vi "rfmapper.vi"() -> ()   [LabVIEW 2011]
uses:
  <instrlib>/niHWS/nihws.llb/niHWS Open File Permissions ID.ctl
  <vilib>/vision/Image Controls.llb/IMAQ Rounding Mode.ctl
  <vilib>/DAQmx/write.llb/DAQmx Write (Analog Wfm 1Chan NSamp).vi
  <vilib>/DAQmx/read.llb/DAQmx Read (Analog 1D Wfm NChan NSamp).vi
  <vilib>/DAQmx/create/channels.llb/DAQmx Create Channel (AO-Voltage-Basic).vi
  <vilib>/DAQmx/configure/timing.llb/DAQmx Timing (Sample Clock).vi
  <vilib>/DAQmx/create/channels.llb/DAQmx Create Channel (AI-Voltage-Basic).vi
  <instrlib>/niHWS/nihws.llb/niHWS Write Analog DBL.vi
  <vilib>/DAQmx/miscellaneous.llb/DAQmx Fill In Error Info.vi
  <vilib>/Analysis/2dsp.llb/1D Cross Correlation (DBL).vi
  <vilib>/Analysis/baseanly.llb/Real Outer Product.vi
  <instrlib>/niHWS/nihws.llb/niHWS Write Analog WDT.vi
  <vilib>/Analysis/NI_AALBase.lvlib
  <vilib>/Analysis/NI_AALPro.lvlib
  <vilib>/ptbypt/NI_PtbyPt.lvlib
  <vilib>/vision/NI_Vision_Development_Module.lvlib
  C:/Program Files/National Instruments/LabVIEW 2011/resource/objmgr/IMAQImage.rc
  C:/Program Files/National Instruments/LabVIEW 2011/resource/objmgr/daqmx.rc
panel:
  in  "Audio Channel":dbl
  out "Waveform Chart 4":dynamicdata(graph)
  in  "audio gain":dbl(knob) scale=0.0..1000000000.0
  in  "Image Size\nX                  Y":dbl[][](array[numeric])=[[0.02, 0.0], [0.99, 0.55]]
  in  "Threshold":dbl=0.3
  in  "Auto\nThreshold":bool
  in  "Recording Path":path
  in  "Record":bool
  in  "Recording channels":tag
  in  "Auto \nDelay":bool
  in  "90-270 delay":dbl
  in  "0-180 delay":dbl
  in  "Ref. \nperiod":dbl=3.0 caption="Time Target (s)"
  out "Count":bool
  out "Wait":bool
  in  "Filter":bool=TRUE
  in  "Binarize Map":bool
  in  "Clear 270":bool
  in  "Clear 180":bool
  in  "Clear 90":bool
  in  "Clear 0":bool
  out "Screen":T1(plugin-control)
  out "Collected Signals 3":dbl[][](graph) caption="Collected Signals"
  out "Waveform Graph":dbl[][](graph)
  out "signal size":i32
  out "270":i32[](array[numeric])
  out "90":i32[](array[numeric])
  out "180":i32[](array[numeric])
  out "0":i32[](array[numeric])
  in  "Bar Direction":u16(ring)=4 items=["270"=3, "90"=2, "180"=1, "0"=0]
  out "Collected Signals 2":dbl[][](graph) caption="Collected Signals"
  out "Waveform Chart 3":dynamicdata(graph)
  out "Collected Signals":dbl[](graph)
  out "Trigger":bool
  out "Waveform Chart":waveform(dbl)(graph)
  in  "stop":bool
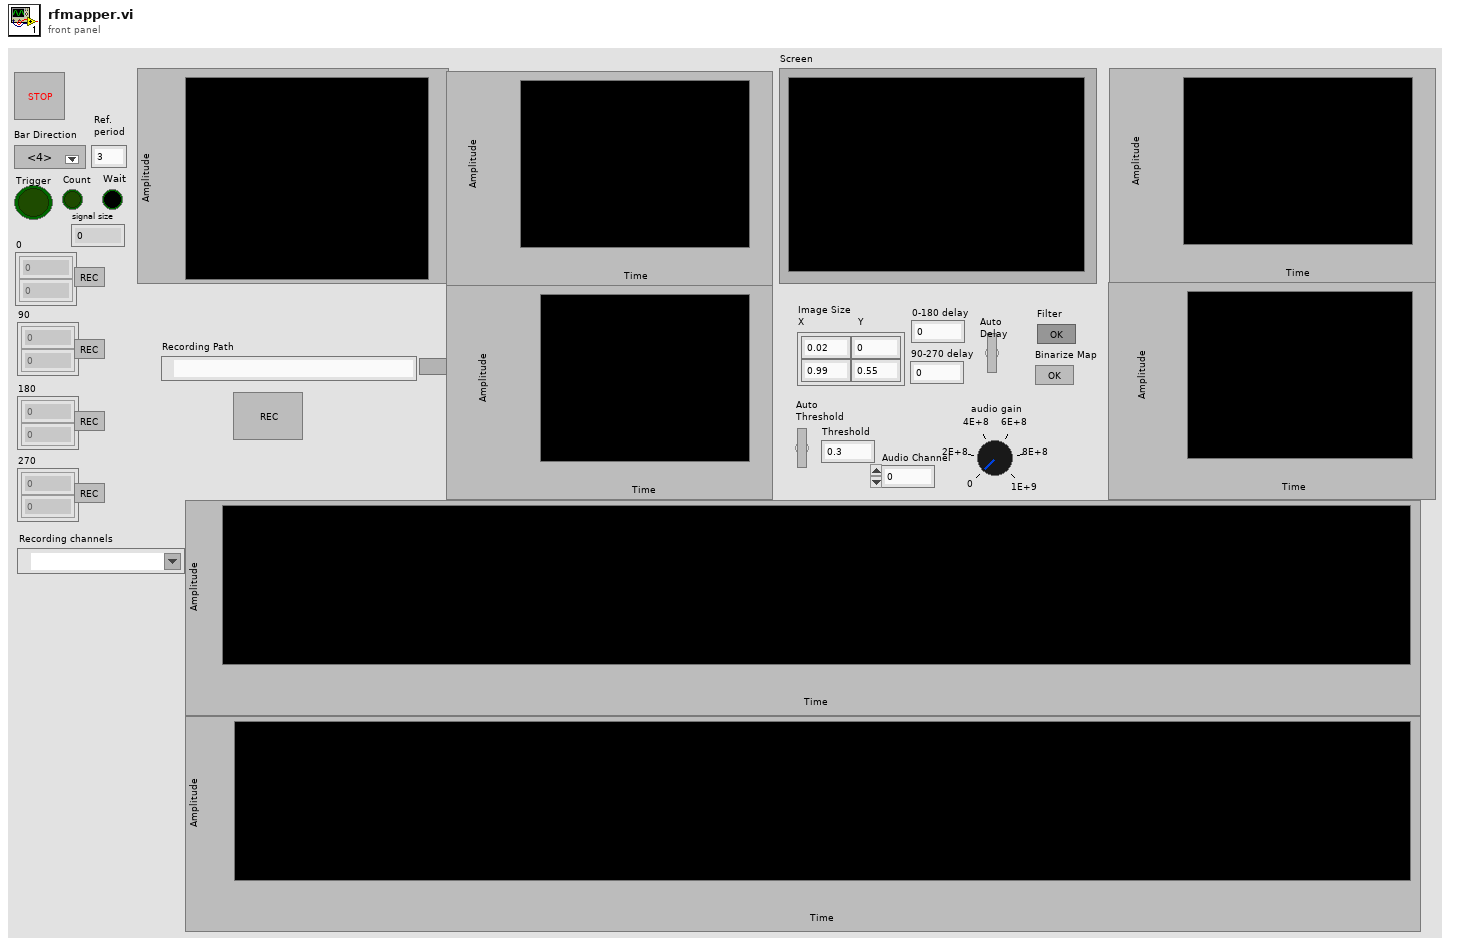
[diagram p1: front panel]
types:
  T1 = typedef "IMAQ Image.ctl" = refnum<image>
  T2 = typedef "niHWS Open File Permissions ID.ctl" = enum32{"Read Only", "Read/Write Existing", "Read/Write/Create New", "Read/Write/Create New Always"}
  T3 = typedef "Image Type" = u32
  T4 = typedef "IMAQ Rounding Mode.ctl" = enum16{"Optimize", "Truncate"}
  T5 = typedef "NI_Matrix.lvlib/RealMatrix.ctl" = dbl[][]
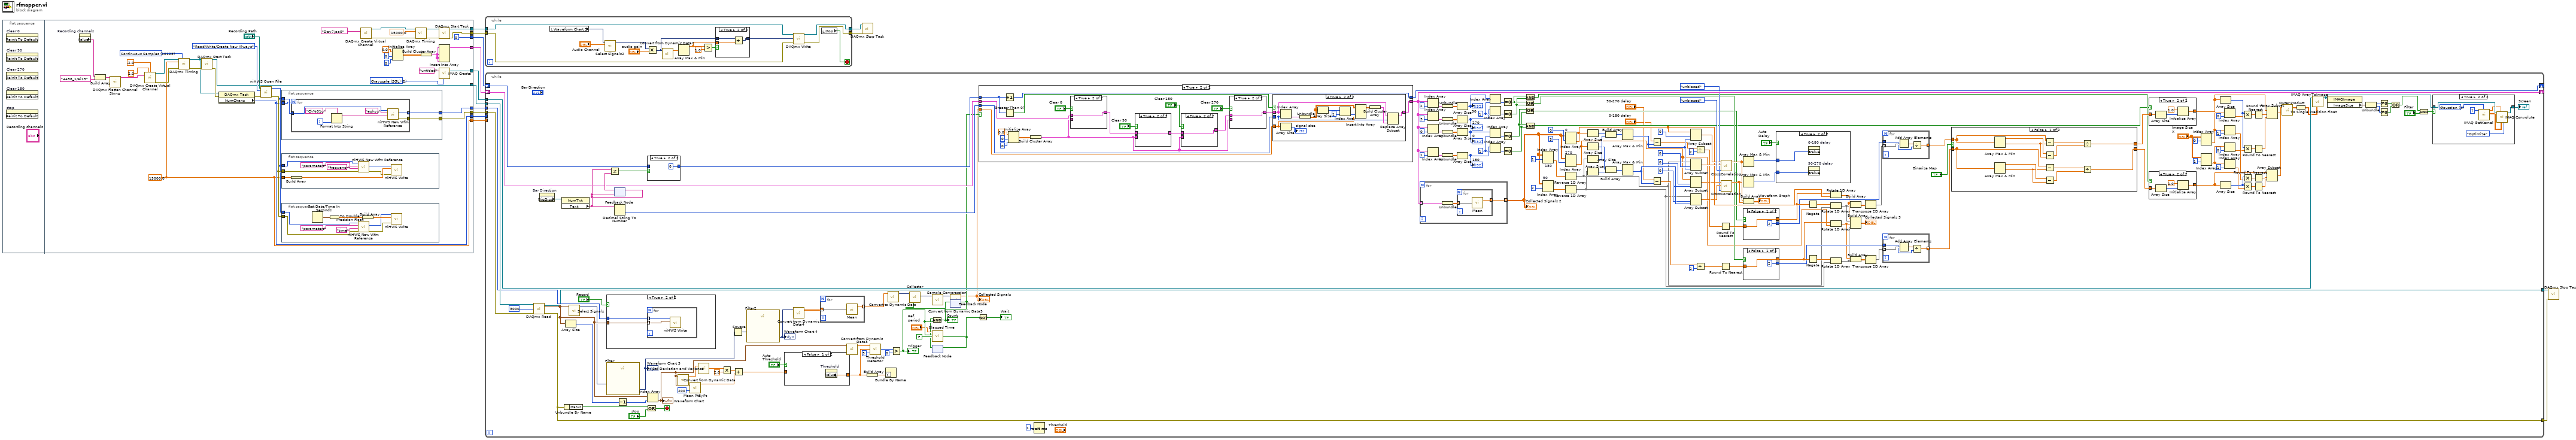
[diagram p0: block diagram]
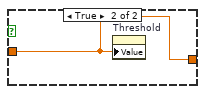
[diagram p3: hidden frame]
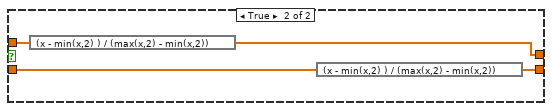
[diagram p7: hidden frame]
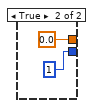
[diagram p10: hidden frame]
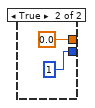
[diagram p11: hidden frame]
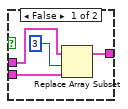
[diagram p14: hidden frame]
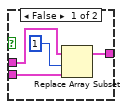
[diagram p15: hidden frame]
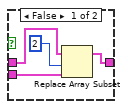
[diagram p16: hidden frame]
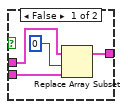
[diagram p17: hidden frame]
diagram:
  n1 = flat-sequence {
    tunnel: [0] -> w14
    tunnel: [w49] -> w13
    tunnel: [w47] -> w12
    tunnel: [w31] -> w11
    tunnel: [w30] -> w10
    tunnel: [w29] -> w9
    tunnel: [w28] -> w8
    tunnel: [w27] -> w5
    tunnel: [w16] -> w2
    tunnel: [w15] -> w1
    frame #0 {
      n2 = invoke on="Clear 0" class="Bool (strict)" method="Reinit To Default"() -> ()  [unwired: 3 in, 3 out]
      n3 = invoke on="Clear 90" class="Bool (strict)" method="Reinit To Default"() -> ()  [unwired: 3 in, 3 out]
      n4 = invoke on="Clear 270" class="Bool (strict)" method="Reinit To Default"() -> ()  [unwired: 3 in, 3 out]
      n5 = invoke on="Clear 180" class="Bool (strict)" method="Reinit To Default"() -> ()  [unwired: 3 in, 3 out]
      n6 = invoke on="stop" class="Bool (strict)" method="Reinit To Default"() -> ()  [unwired: 3 in, 3 out]
    }
    frame #1 {
      w41 = 10123 items=["Finite Samples"=10178, "Continuous Samples"=10123, "Hardware Timed Single Point"=12522] ("sample mode")
      w27 = 15000.0 ("rate")
      w45 = T3 2 items=["Grayscale (U8)", "Grayscale (I16)", "Grayscale (SGL)", "Complex (CSG)", "RGB (U32)", "HSL (U32)", "RGB (U64)", "Grayscale (U16)"] ("Image Type")
      n7 = property on="Recording channels" class="DAQmxName"() -> ("Value"=w24:string)  [unwired: 2 in, 2 out]
      n8 = Build Array(w24, tag "4498_1/ai15" ("Recording channels 3")) -> (w26:string[])
      n9 = call <vilib>:"DAQmx Flatten Channel String.vi"("names in"=w26) -> ("names out"=w23:string)  [unwired: 13 in, 1 out]
      n10 = call-poly <vilib>:"DAQmx Create Virtual Channel.vi"("maximum value"=2.0, "minimum value"=-2.0, "physical channels"=w23) -> ("task out"=w42:refnum<k21>, "error out"=w40:errorcluster)  [unwired: 11 in]
      n11 = call-poly <vilib>:"DAQmx Timing.vi"("task/channels in"=w42, "sample mode"=w41, "rate"=w27, "error in"=w40) -> ("task out"=w37:refnum<k21>, "error out"=w39:errorcluster)  [unwired: 10 in]
      n12 = call <vilib>:"DAQmx Start Task.vi"("task/channels in"=w37, "error in"=w39) -> ("task out"=w31:refnum<k21>, "error out"=w38:errorcluster)  [unwired: 12 in]
      n13 = property class="DAQmx Task"(reference=w37, error in=w38) -> (error out=w34:errorcluster, "NumChans"=w30:u32)  [unwired: 1 out]
      n14 = call <instrlib>:"niHWS Open File.vi"("error in (no error)"=w34, "permissions (0:read only)"=niHWS_Open_File_Permissions_ID."Read/Write/Create New Always", "file path"="Recording Path") -> ("error out"=w33:errorcluster, "file handle"=w32:u32)  [unwired: 7 in]
      n15 = flat-sequence {
        tunnel: w30 -> [w74]
        tunnel: w32 -> [w75]
        tunnel: [w73] -> w28
        tunnel: [w72] -> w29
        frame #0 {
          n16 = for {
            N: w74 -> [_]
            tunnel: [w77] -> w73 mode=indexing
            tunnel: [w76] -> w72
            tunnel: w75 -> [w82]
            i -> [w80]
            n17 = Format Into String(format string="Ch%01u", w80) -> (resulting string=w78:string)  [unwired: 2 in, 1 out]
            n18 = call <instrlib>:"niHWS New Wfm Reference.vi"("waveform name (empty)"=w78, "group name (empty)"="ephys", "file handle in"=w82) -> ("error out"=w76:errorcluster, "waveform reference"=w77:u32)  [unwired: 6 in, 1 out]
          }
        }
      }
      n19 = flat-sequence {
        tunnel: w27 -> [w67]
        tunnel: w33 -> [w66]
        tunnel: w32 -> [w65]
        frame #0 {
          n20 = Build Array(w67) -> (w68:dbl[])
          n21 = call <instrlib>:"niHWS New Wfm Reference.vi"("error in (no error)"=w66, "waveform name (empty)"="frequency" ("group name (empty)"), "group name (empty)"="parameters", "file handle in"=w65) -> ("error out"=w64:errorcluster, "waveform reference"=w71:u32)  [unwired: 5 in, 1 out]
          n22 = call-poly <instrlib>:"niHWS Write.vi"("error in (no error)"=w64, "data"=w68, "waveform reference in"=w71) -> ()  [unwired: 7 in, 2 out]
        }
      }
      n23 = flat-sequence {
        tunnel: w33 -> [w63]
        tunnel: w32 -> [w62]
        frame #0 {
          n24 = Get Date/Time In Seconds() -> (seconds since 1Jan1904=w61:timestamp)
          n25 = To Double Precision Float(number=w61) -> (double precision float=w60:dbl)
          n26 = call <instrlib>:"niHWS New Wfm Reference.vi"("error in (no error)"=w63, "waveform name (empty)"="time" ("group name (empty)"), "group name (empty)"="parameters", "file handle in"=w62) -> ("error out"=w55:errorcluster, "waveform reference"=w56:u32)  [unwired: 5 in, 1 out]
          n27 = Build Array(w60) -> (w59:dbl[])
          n28 = call-poly <instrlib>:"niHWS Write.vi"("error in (no error)"=w55, "data"=w59, "waveform reference in"=w56) -> ()  [unwired: 7 in, 2 out]
        }
      }
      n29 = call-poly <vilib>:"DAQmx Create Virtual Channel.vi"("physical channels"=tag "Dev7/ao0") -> ("task out"=w21:refnum<k21>, "error out"=w18:errorcluster)  [unwired: 13 in]
      n30 = Initialize Array(0.0, 0, 0) -> (w53:dbl[][])
      n31 = call-poly <vilib>:"DAQmx Timing.vi"("task/channels in"=w21, "rate"=15000.0, "error in"=w18) -> ("task out"=w19:refnum<k21>, "error out"=w17:errorcluster)  [unwired: 11 in]
      n32 = Build Cluster Array(w53) -> (w48:cluster{dbl[][]}[])
      n33 = call <vilib>:"DAQmx Start Task.vi"("task/channels in"=w19, "error in"=w17) -> ("task out"=w16:refnum<k21>, "error out"=w15:errorcluster)  [unwired: 12 in]
      n34 = Insert Into Array(array=w48, new element #1=w48, new element #2=w48, new element #3=w48) -> (w49:cluster{dbl[][]}[])  [unwired: 1 in]
      n35 = call "IMAQ Create"("Image Name"="untitled", "Image Type"=w45) -> ("New Image"=w47:T1)  [unwired: 3 in, 1 out]
    }
  }
  n36 = while {
    tunnel: [w96] -> w4
    tunnel: [w95] -> w3
    tunnel: w2 -> [w94]
    tunnel: w1 -> [w93]
    stop <- w97 stop-if-true
    n37 = local read "Waveform Chart 3"() -> (w85:dynamicdata)
    n38 = call "Select Signals2"("Selector Input"="Audio Channel", "Signals"=w85) -> ("Signal Out"=w83:dynamicdata)  [unwired: 8 in, 1 out]
    n39 = Multiply(x=w83, y="audio gain") -> (x*y=w88:dynamicdata)
    n40 = call "Convert from Dynamic Data2"("Dynamic Data Type"=w88) -> ("Array"=w91:dbl[])  [unwired: 3 in]
    n41 = Array Max & Min(array=w91) -> (max value=w86:dbl)  [unwired: 3 out]
    n42 = Greater?(x=w86, y=1.0) -> (0:w89:bool)
    n43 = case shown="True" w89 {
      tunnel: w88 -> [w98 w101]
      tunnel: [w98 w99] -> w87
      tunnel: w86 -> [_ w100]
      frame False {
      }
      frame True {
        n44 = Divide(x=w101, y=w100) -> (x/y=w99:dynamicdata)
      }
    }
    n45 = call-poly <vilib>:"DAQmx Write.vi"("task/channels in"=w94, "data"=w87, "error in"=w93) -> ("task out"=w96:refnum<k21>, "error out"=w95:errorcluster)  [unwired: 10 in, 1 out]
    n46 = local read "stop"() -> (w97:bool)
  }
  n47 = while {
    shift-right: [w285] -> _
    shift-left: w14 -> [w264]
    shift-right: [w271] -> _
    shift-left: w13 -> [w201]
    tunnel: w12 -> [w209]
    tunnel: w11 -> [w164]
    tunnel: w10 -> [_]
    tunnel: w9 -> [w165]
    tunnel: w8 -> [w163]
    tunnel: [w158] -> w7
    tunnel: [w157] -> w6
    tunnel: w5 -> [_]
    stop <- w159 stop-if-true
    w220 = 1 ("index")
    w227 = 1 ("index")
    n48 = call-poly <vilib>:"DAQmx Read.vi"("task/channels in"=w164, "number of samples per channel"=3000, "error in"=w165) -> ("task out"=w158:refnum<k21>, "data"=w129:waveform(dbl)[], "error out"=w157:errorcluster)  [unwired: 10 in]
    n49 = property on="Bar Direction" class="Ring (strict)"() -> ("DigDisp"=w284:refnum<vi>)  [unwired: 2 in, 2 out]
    n50 = property class="NumTxt"(reference=w284) -> ("Text"=w266:string)  [unwired: 1 in, 2 out]
    n51 = Unbundle By Name(w157) -> ("status"=w161:bool)
    n52 = Array Size(array=w129) -> (size(s)=w131:i32)
    n53 = call "Select Signals"("Signals"=w129) -> ("Signal Out"=w124:dynamicdata)  [unwired: 9 in, 1 out]
    n54 = case shown="True" "Record" {
      tunnel: w129 -> [_ w299]
      tunnel: w163 -> [_ w298]
      frame False {
      }
      frame True {
        n55 = for {
          tunnel: w299 -> [w301] mode=indexing
          tunnel: w298 -> [w300] mode=indexing
          n56 = call-poly <instrlib>:"niHWS Write.vi"("analog waveform"=w301, "waveform reference in"=w300) -> ()  [unwired: 8 in, 2 out]
        }
      }
    }
    n57 = call "Filter"("Signal"=w124) -> ("Filtered Signal"=w102:dynamicdata)  [unwired: 9 in, 1 out]
    "Waveform Chart 3" <- w102
    n58 = feedback-in #1(w266) -> ()
    n59 = feedback #1(w266) -> (w265:string)
    n60 = Not Equal?(x=w266, y=w265) -> (x != y?=w262:bool)
    n61 = Decimal String To Number(string=w266) -> (number=w270:i32)  [unwired: 2 in, 1 out]
    n62 = Decrement(x=w131) -> (x-1=w130:i32)
    n63 = Or(x=w161, y="stop") -> (x .or. y?=w159:bool)
    n64 = case shown="True" w262 {
      tunnel: w264 -> [w354 _]
      tunnel: [w354 0] -> w263
      frame False {
      }
      frame True {
      }
    }
    n65 = Index Array(array=w129, index=w130) -> (element=w123:waveform(dbl))
    "Waveform Chart" <- w123
    n66 = call "Convert from Dynamic Data"("Dynamic Data Type"=w123) -> ("Array"=w292:dbl[])  [unwired: 3 in]
    n67 = call <vilib>:"Mean PtByPt.vi"("x"=w123, "sample length"=200) -> ("mean"=w287:dbl)  [unwired: 2 in, 1 out]
    n68 = call <vilib>:"Std Deviation and Variance.vi"("X"=w292) -> ("standard deviation"=w291:dbl)  [unwired: 1 in, 2 out]
    n69 = Multiply(x=w291, y=2.0) -> (x*y=w288:dbl)
    n70 = Square(x=w102) -> (x^2=w104:dynamicdata)
    n71 = Add(x=w288, y=w287) -> (x+y=w152:dbl)
    n72 = call "Filter2"("Signal"=w104) -> ("Filtered Signal"=w103:dynamicdata)  [unwired: 9 in, 1 out]
    "Waveform Chart 4" <- w103
    n73 = case shown="False" "Auto\nThreshold" {
      tunnel: w152 -> [_ w297]
      tunnel: [w296 w297] -> w151
      frame False {
        n74 = property on="Threshold" class="DigNum (strict)"() -> ("Value"=w296:dbl)  [unwired: 2 in, 2 out]
      }
      frame True {
        n75 = property on="Threshold" class="DigNum (strict)"("Value"=w297) -> ()  [unwired: 2 in, 2 out]
      }
    }
    n76 = call "Convert from Dynamic Data4"("Dynamic Data Type"=w103) -> ("Array"=w128:dbl[][])  [unwired: 3 in]
    n77 = for {
      tunnel: w128 -> [w295] mode=indexing
      tunnel: [w294] -> w127 mode=indexing
      n78 = call <vilib>:"Mean.vi"("X"=w295) -> ("mean"=w294:dbl)  [unwired: 1 out]
    }
    n79 = call "Convert from Dynamic Data3"("Dynamic Data Type"=w123) -> ("Array"=w290:dbl[])  [unwired: 3 in]
    n80 = Build Array(w151) -> (w150:dbl[])
    n81 = call <vilib>:"Threshold Detector.vi"("width"=3, "threshold"=w151, "X"=w290) -> ("count"=w286:i32)  [unwired: 2 out]
    n82 = Bundle By Name("Y"=w150) -> ()  [unwired: 1 in, 1 out]
    n83 = call "Convert to Dynamic Data"("Array"=w127) -> ("Dynamic Data Type"=w126:dynamicdata)  [unwired: 3 in]
    n84 = Greater?(x=w286, y=0) -> (0:w177:bool)
    "Trigger" <- w177
    n85 = call "Elapsed Time"("Time Target (s)"="Ref. \nperiod", "Reset"=w177, "Auto Reset"=FALSE) -> ("Time has Elapsed"=w173:bool)  [unwired: 9 in, 7 out]
    n86 = feedback-in #2(w173) -> ()
    n87 = feedback #2() -> (w174:bool)  [unwired: 1 in]
    n88 = And(x=w174, y=w177) -> (x .and. y?=w133:bool)
    "Count" <- w133
    n89 = feedback-in #3(w133) -> ()
    n90 = feedback #3() -> (w132:bool)  [unwired: 1 in]
    n91 = call "Collector"("Reset"=w132, "Signals"=w126) -> ("Collected Signals"=w106:dynamicdata)  [unwired: 8 in, 1 out]
    n92 = call "Sample Compression"("Signals"=w106) -> ("Mean"=w105:dynamicdata)  [unwired: 8 in, 2 out]
    n93 = call "Convert from Dynamic Data5"("Dynamic Data Type"=w105) -> ("Array"=w125:dbl[])  [unwired: 3 in]
    "Collected Signals" <- w125
    n94 = Not(x=w173) -> (.not. x?=→"Wait":bool)
    n95 = case shown="True" w133 {
      tunnel: w263 -> [w362 w379]
      tunnel: [w362 w382] -> w285
      tunnel: w201 -> [w361 w373]
      tunnel: w125 -> [_ w363]
      tunnel: [w361 w381] -> w271
      tunnel: w270 -> [_ w380]
      frame False {
      }
      frame True {
        n96 = Increment(x=w379) -> (x+1=w382:i32)
        n97 = Greater Than 0?(x=w379) -> (x > 0?=w378:bool)
        n98 = Initialize Array(0.0, 0, 0) -> (w377:dbl[][])
        n99 = Build Cluster Array(w377) -> (w372:cluster{dbl[][]}[])
        n100 = case shown="True" "Clear 0" {
          tunnel: w373 -> [w400 w402]
          tunnel: [w398 w402] -> w364
          tunnel: w372 -> [w399 _]
          frame False {
            n101 = Replace Array Subset(array=w400, new element=w399, index=0) -> (w398:cluster{dbl[][]}[])
          }
          frame True {
          }
        }
        n102 = case shown="True" "Clear 90" {
          tunnel: w364 -> [w395 w397]
          tunnel: w372 -> [w394 _]
          tunnel: [w393 w397] -> w371
          frame False {
            n103 = Replace Array Subset(array=w395, new element=w394, index=2) -> (w393:cluster{dbl[][]}[])
          }
          frame True {
          }
        }
        n104 = case shown="True" "Clear 180" {
          tunnel: w371 -> [w390 w392]
          tunnel: w372 -> [w389 _]
          tunnel: [w388 w392] -> w370
          frame False {
            n105 = Replace Array Subset(array=w390, new element=w389, index=1) -> (w388:cluster{dbl[][]}[])
          }
          frame True {
          }
        }
        n106 = case shown="True" "Clear 270" {
          tunnel: w370 -> [w385 w387]
          tunnel: [w384 w387] -> w369
          tunnel: w372 -> [w383 _]
          frame False {
            n107 = Replace Array Subset(array=w385, new element=w383, index=3) -> (w384:cluster{dbl[][]}[])
          }
          frame True {
          }
        }
        n108 = case shown="True" w378 {
          tunnel: [w403 w415] -> w381
          tunnel: w380 -> [_ w412]
          tunnel: w363 -> [_ w407]
          tunnel: w369 -> [w403 w404]
          frame False {
          }
          frame True {
            n109 = Index Array(array=w404, index=w412) -> (element=w413:cluster{dbl[][]})
            n110 = Array Size(array=w407) -> (size(s)=→"signal size":i32)
            n111 = Unbundle(w413) -> (w411:dbl[][])
            n112 = Array Size(array=w411) -> (size(s)=w410:i32[])
            n113 = Index Array(array=w410, index=1) -> (element=w408:i32)
            n114 = Insert Into Array(array=w411, index (col)=w408, new element=w407) -> (w405:dbl[][])  [unwired: 1 in]
            n115 = Build Cluster Array(w405) -> (w414:cluster{dbl[][]}[])
            n116 = Replace Array Subset(array=w404, new element=w414, index=w412) -> (w415:cluster{dbl[][]}[])
          }
        }
      }
    }
    n117 = Wait (ms)(milliseconds to wait=u32 1) -> ()  [unwired: 1 out]
    n118 = for {
      tunnel: [w358] -> w231 mode=indexing
      tunnel: w271 -> [w357] mode=indexing
      n119 = Unbundle(w357) -> (w356:dbl[][])
      n120 = for {
        tunnel: [w359] -> w358 mode=indexing
        tunnel: w356 -> [w360] mode=indexing
        n121 = call <vilib>:"Mean.vi"("X"=w360) -> ("mean"=w359:dbl)  [unwired: 1 out]
      }
    }
    "Collected Signals 2" <- w231
    n122 = Index Array(array=w271, index=2) -> (element=w277:cluster{dbl[][]})
    n123 = Index Array(array=w271, index=3) -> (element=w279:cluster{dbl[][]})
    n124 = Index Array(array=w271, index=0) -> (element=w273:cluster{dbl[][]})
    n125 = Index Array(array=w271, index=1) -> (element=w275:cluster{dbl[][]})
    n126 = Unbundle(w277) -> (w276:dbl[][])
    n127 = Unbundle(w279) -> (w278:dbl[][])
    n128 = Unbundle(w273) -> (w272:dbl[][])
    n129 = Unbundle(w275) -> (w274:dbl[][])
    n130 = Array Size(array=w276) -> (size(s)=w219:i32[])
    "90" <- w219
    n131 = Array Size(array=w278) -> (size(s)=w218:i32[])
    "270" <- w218
    n132 = Array Size(array=w272) -> (size(s)=w229:i32[])
    "0" <- w229
    n133 = Array Size(array=w274) -> (size(s)=w228:i32[])
    "180" <- w228
    n134 = Index Array(array=w219, index=w220) -> (element=w221:i32)
    n135 = Index Array(array=w218, index=w220) -> (element=w222:i32)
    n136 = Index Array(array=w229, index=w227) -> (element=w226:i32)
    n137 = Index Array(array=w228, index=w227) -> (element=w225:i32)
    n138 = Equal To 0?(x=w221) -> (x = 0?=w196:bool)
    n139 = Equal To 0?(x=w222) -> (x = 0?=w195:bool)
    n140 = Equal To 0?(x=w226) -> (x = 0?=w194:bool)
    n141 = Equal To 0?(x=w225) -> (x = 0?=w193:bool)
    n142 = Or(x=w196, y=w195) -> (x .or. y?=w200:bool)
    n143 = Or(x=w194, y=w193) -> (x .or. y?=w197:bool)
    n144 = And(x=w196, y=w195) -> (x .and. y?=w192:bool)
    n145 = And(x=w194, y=w193) -> (x .and. y?=w191:bool)
    n146 = Index Array "180"(array=w231, index (row)=1) -> (element=w147:dbl[])  [unwired: 1 in]
    n147 = Index Array "90"(array=w231, index (row)=2) -> (element=w149:dbl[])  [unwired: 1 in]
    n148 = Index Array "0"(array=w231, index (row)=0) -> (element=w252:dbl[])  [unwired: 1 in]
    n149 = Index Array "270"(array=w231, index (row)=3) -> (element=w134:dbl[])  [unwired: 1 in]
    n150 = Reverse 1D Array(array=w147) -> (reversed array=w148:dbl[])
    n151 = Reverse 1D Array(array=w149) -> (reversed array=w135:dbl[])
    n152 = Array Size(array=w252) -> (size(s)=w257:i32)
    n153 = Array Size(array=w134) -> (size(s)=w237:i32)
    n154 = Array Size(array=w148) -> (size(s)=w256:i32)
    n155 = Array Size(array=w135) -> (size(s)=w238:i32)
    n156 = Build Array(w257, w256) -> (w255:i32[])
    n157 = Build Array(w237, w238) -> (w239:i32[])
    n158 = Array Max & Min(array=w255) -> (min value=w248:i32)  [unwired: 3 out]
    n159 = Array Max & Min(array=w239) -> (min value=w245:i32)  [unwired: 3 out]
    n160 = Subtract(x="0-180 delay", y=w248) -> (x-y=w247:dbl)
    n161 = Subtract(x="90-270 delay", y=w245) -> (x-y=w246:dbl)
    n162 = Array Subset(array=w252, index=0, length=w248) -> (w254:dbl[])
    n163 = Array Subset(array=w148, index=0, length=w248) -> (w253:dbl[])
    n164 = Array Subset(array=w134, index=0, length=w245) -> (w240:dbl[])
    n165 = Array Subset(array=w135, index=0, length=w245) -> (w241:dbl[])
    n166 = Divide(x=w247, y=2) -> (x/y=w249:dbl)
    n167 = Divide(x=w246, y=2) -> (x/y=w244:dbl)
    n168 = Round To Nearest(number=w249) -> (nearest integer value=w224:dbl)
    n169 = Round To Nearest(number=w244) -> (nearest integer value=w217:dbl)
    n170 = call-poly <vilib>:"CrossCorrelation.vi"("normalization"=enum32{"none", "unbiased", "biased"}."unbiased", "Y"=w253, "X"=w254) -> ("Rxy"=w260:dbl[])  [unwired: 7 in, 1 out]
    n171 = call-poly <vilib>:"CrossCorrelation.vi"("normalization"=enum32{"none", "unbiased", "biased"}."unbiased", "Y"=w241, "X"=w240) -> ("Rxy"=w230:dbl[])  [unwired: 7 in, 1 out]
    n172 = Array Max & Min(array=w260) -> (max index (indices)=w169:i32)  [unwired: 3 out]
    n173 = Array Max & Min(array=w230) -> (max index (indices)=w170:i32)  [unwired: 3 out]
    n174 = Build Array(w260, w230) -> (→"Waveform Graph":dbl[][])
    n175 = case shown="False" w197 {
      tunnel: [w351 0.0] -> w223
      tunnel: w224 -> [w351 _]
      tunnel: [2 1] -> w211
      frame False {
      }
      frame True {
      }
    }
    n176 = case shown="False" w200 {
      tunnel: [w347 0.0] -> w216
      tunnel: w217 -> [w347 _]
      tunnel: [2 1] -> w210
      frame False {
      }
      frame True {
      }
    }
    n177 = case shown="True" "Auto \nDelay" {
      tunnel: w170 -> [_ w303]
      tunnel: w169 -> [_ w302]
      frame False {
      }
      frame True {
        n178 = property on="0-180 delay" class="DigNum (strict)"("Value"=w302) -> ()  [unwired: 2 in, 2 out]
        n179 = property on="90-270 delay" class="DigNum (strict)"("Value"=w303) -> ()  [unwired: 2 in, 2 out]
      }
    }
    n180 = Negate(x=w223) -> (-x=w251:dbl)
    n181 = Negate(x=w216) -> (-x=w242:dbl)
    n182 = Rotate 1D Array(1:w252, 2:w223) -> (0:w205:dbl[])
    n183 = Rotate 1D Array(1:w148, 2:w251) -> (0:w204:dbl[])
    n184 = Rotate 1D Array(1:w134, 2:w216) -> (0:w203:dbl[])
    n185 = Rotate 1D Array(1:w135, 2:w242) -> (0:w202:dbl[])
    n186 = Build Array(w205, w204) -> (w213:dbl[][])
    n187 = Build Array(w205, w204, w203, w202) -> (→"Collected Signals 3":dbl[][])
    n188 = Build Array(w203, w202) -> (w215:dbl[][])
    n189 = Transpose 2D Array(2D array=w213) -> (transposed array=w212:dbl[][])
    n190 = Transpose 2D Array(2D array=w215) -> (transposed array=w214:dbl[][])
    n191 = for {
      tunnel: [w345] -> w208 mode=indexing
      tunnel: w212 -> [w343] mode=indexing
      tunnel: w211 -> [w342]
      n192 = Add Array Elements(numeric array=w343) -> (sum=w344:dbl)
      n193 = Divide(x=w344, y=w342) -> (x/y=w345:dbl)
    }
    n194 = for {
      tunnel: [w340] -> w206 mode=indexing
      tunnel: w214 -> [w339] mode=indexing
      tunnel: w210 -> [w338]
      n195 = Add Array Elements(numeric array=w339) -> (sum=w341:dbl)
      n196 = Divide(x=w341, y=w338) -> (x/y=w340:dbl)
    }
    n197 = case shown="False" "Binarize Map" {
      tunnel: w208 -> [w315 w327]
      tunnel: w206 -> [w312 w326]
      tunnel: [w321 w325] -> w199
      tunnel: [w320 w324] -> w198
      frame False {
        n198 = Array Max & Min(array=w315) -> (max value=w317:dbl, min value=w316:dbl)  [unwired: 2 out]
        n199 = Array Max & Min(array=w312) -> (max value=w314:dbl, min value=w313:dbl)  [unwired: 2 out]
        n200 = Subtract(x=w315, y=w316) -> (x-y=w319:dbl[])
        n201 = Subtract(x=w317, y=w316) -> (x-y=w318:dbl)
        n202 = Subtract(x=w312, y=w313) -> (x-y=w323:dbl[])
        n203 = Subtract(x=w314, y=w313) -> (x-y=w322:dbl)
        n204 = Divide(x=w319, y=w318) -> (x/y=w320:dbl[])
        n205 = Divide(x=w323, y=w322) -> (x/y=w321:dbl[])
      }
      frame True {
        n206 = expression code="(x - min(x,2) ) / (max(x,2) - min(x,2))"(w327) -> (w324:dbl[])
        n207 = expression code="(x - min(x,2) ) / (max(x,2) - min(x,2))"(w326) -> (w325:dbl[])
      }
    }
    n208 = case shown="True" w191 {
      tunnel: w198 -> [w328 w332]
      tunnel: [w328 w329] -> w122
      frame False {
      }
      frame True {
        n209 = Array Size(array=w332) -> (size(s)=w331:i32)
        n210 = Initialize Array(1.0 ("element"), w331) -> (w329:dbl[])
      }
    }
    n211 = case shown="True" w192 {
      tunnel: w199 -> [w333 w337]
      tunnel: [w333 w334] -> w121
      frame False {
      }
      frame True {
        n212 = Array Size(array=w337) -> (size(s)=w336:i32)
        n213 = Initialize Array(1.0 ("element"), w336) -> (w334:dbl[])
      }
    }
    n214 = Index Array(array="Image Size\nX                  Y", index (row)=0) -> (element=w141:dbl[])  [unwired: 1 in]
    n215 = Index Array(array="Image Size\nX                  Y", index (row)=1) -> (element=w140:dbl[])  [unwired: 1 in]
    n216 = Array Size(array=w122) -> (size(s)=w111:i32)
    n217 = Array Size(array=w121) -> (size(s)=w116:i32)
    n218 = Index Array(array=w141, index=0) -> (element=w107:dbl)
    n219 = Index Array(array=w141, index=1) -> (element=w115:dbl)
    n220 = Index Array(array=w140, index=0) -> (element=w110:dbl)
    n221 = Index Array(array=w140, index=1) -> (element=w112:dbl)
    n222 = Multiply(x=w111, y=w107) -> (x*y=w120:dbl)
    n223 = Multiply(x=w111, y=w110) -> (x*y=w119:dbl)
    n224 = Multiply(x=w116, y=w115) -> (x*y=w118:dbl)
    n225 = Multiply(x=w116, y=w112) -> (x*y=w117:dbl)
    n226 = Round To Nearest(number=w120) -> (nearest integer value=w108:dbl)
    n227 = Round To Nearest(number=w119) -> (nearest integer value=w109:dbl)
    n228 = Round To Nearest(number=w118) -> (nearest integer value=w114:dbl)
    n229 = Round To Nearest(number=w117) -> (nearest integer value=w113:dbl)
    n230 = Array Subset(array=w122, index=w108, length=w109) -> (w145:dbl[])
    n231 = Array Subset(array=w121, index=w114, length=w113) -> (w146:dbl[])
    n232 = call-poly <vilib>:"Outer Product.vi"("Y Vector"=w145, "X Vector"=w146) -> ("Outer Product"=w189:T5)  [unwired: 1 out]
    n233 = To Single Precision Float(number=w189) -> (single precision float=w188:sgl[][])
    n234 = call "IMAQ ArrayToImage"("Image Pixels (Float)"=w188, "Image"=w209) -> ("Image Out"=w186:T1)  [unwired: 8 in, 1 out]
    n235 = property class="IMAQImage"(reference=w186) -> ("ImageSize"=w185:cluster{"x":i32, "y":i32})  [unwired: 1 in, 2 out]
    n236 = Unbundle(w185) -> ("x"=w182:i32, "y"=w181:i32)
    n237 = Not Equal To 0?(x=w182) -> (x != 0?=w184:bool)
    n238 = Not Equal To 0?(x=w181) -> (x != 0?=w183:bool)
    n239 = Or(x=w184, y=w183) -> (x .or. y?=w178:bool)
    n240 = And(x=w178, y="Filter") -> (x .and. y?=w180:bool)
    n241 = case shown="True" w180 {
      tunnel: w186 -> [w304 w311]
      tunnel: [w304 w310] -> w187
      frame False {
      }
      frame True {
        w308 = u16 4 items=["Gradient"=1, "Laplacian"=2, "Smoothing"=3, "Gaussian"=4] ("Kernel Family")
        n242 = call "IMAQ GetKernel"("Kernel Family"=w308, "Kernel Size (3,5,...)"=7) -> ("Kernel"=w306:sgl[][], "Divider"=w307:sgl)  [unwired: 6 in, 2 out]
        n243 = call "IMAQ Convolute"("Rounding Mode"=IMAQ_Rounding_Mode."Optimize", "Kernel"=w306, "Divider (kernel sum)"=w307, "Image Src"=w311) -> ("Image Dst Out"=w310:T1)  [unwired: 6 in, 1 out]
      }
    }
    "Screen" <- w187
  }
  n244 = call <vilib>:"DAQmx Stop Task.vi"("task/channels in"=w4, "error in"=w3) -> ()  [unwired: 12 in, 2 out]
  n245 = call <vilib>:"DAQmx Stop Task.vi"("task/channels in"=w7, "error in"=w6) -> ()  [unwired: 12 in, 2 out]
